vi "Inverse Time Curves (Formula, Dependent Reset).vi"(6 "operate time compensation":cluster{"G/Gs":dbl, "compensation [s]":dbl}[](array[cluster]), 7 "GD (25)":u16=25, 8 "error in (no error)":errorcluster, 9 "reset time parameters":T2={"tr [s]"=1.0, "alpha"=1.0}, 10 "time multiplier setting (1)":dbl=1.0, 11 "operate time parameters":T1={"A [s]"=1.0, "B [s]"=1.0, "alpha"=1.0, "K2 [s]"=1.0, "K1 [s]"=1.0, "K3 [s]"=1.0}) -> (0 "error out":errorcluster, 2 "memory size":u16, 3 "memory initial values":fxp<+,51,51>[](array[numeric]), 4 "curve data":cluster{"G/Gs":dbl[], "times [s]":dbl[]})   [LabVIEW 2014, in "NI_EP_Protection.lvlib"]
doc: "Generates memory initial values and memory size, which contain the information of the inverse time curves, for the FPGA Inverse Time Delay VI to use. You can compensate for the processing delay of the input energizing quantity under a specific G/Gs to achieve higher operate time accuracy."
uses:
  <vilib>/addons/Electrical Power/Protection/NI_EP_Protection.lvlib
  <vilib>/addons/Electrical Power/Protection/Inverse Time Delay/subVIs/ep_Reset Time.ctl
  <vilib>/addons/Electrical Power/Protection/Inverse Time Delay/subVIs/ep_Operate Time.ctl
  <vilib>/addons/Electrical Power/Protection/Inverse Time Delay/subVIs/ep_Curve Parameters.ctl
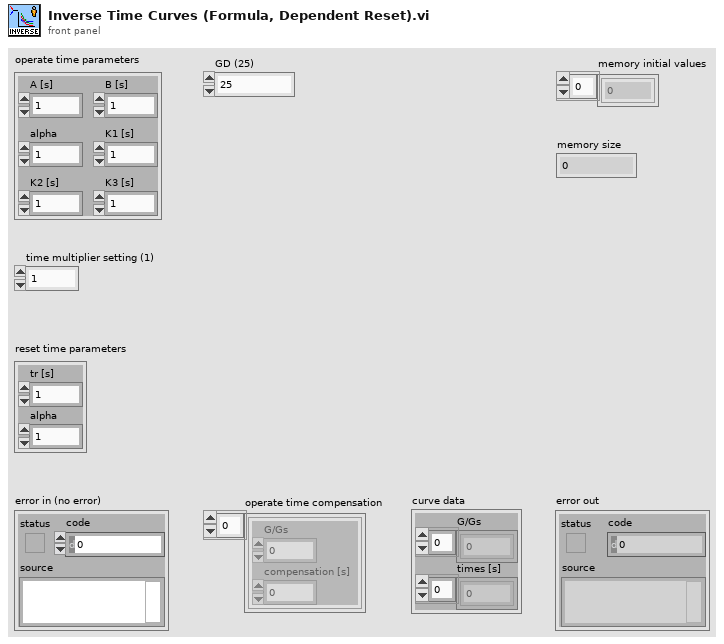
[diagram p1: front panel]
types:
  T1 = typedef "NI_EP_Protection.lvlib/ep_Operate Time.ctl" = cluster{"A [s]":dbl, "B [s]":dbl, "alpha":dbl, "K2 [s]":dbl, "K1 [s]":dbl, "K3 [s]":dbl}
  T2 = typedef "NI_EP_Protection.lvlib/ep_Reset Time.ctl" = cluster{"tr [s]":dbl, "alpha":dbl}
  T3 = typedef "NI_EP_Protection.lvlib/ep_Curve Parameters.ctl" = cluster{"operate time parameters":T1, "reset time parameters":T2}
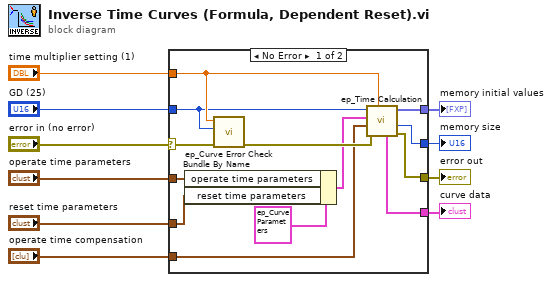
[diagram p0: block diagram]
diagram:
  n1 = case shown="No Error" "error in (no error)" {
    selector: "error in (no error)" -> [w22 w24]
    tunnel: "GD (25)" -> [w21 _]
    tunnel: "time multiplier setting (1)" -> [w23 _]
    tunnel: "operate time parameters" -> [w15 _]
    tunnel: "reset time parameters" -> [w14 _]
    tunnel: [w18 _] -> w7
    tunnel: [w19 _] -> w6
    tunnel: [w17 w24] -> w4
    tunnel: [w16 _] -> w3
    tunnel: "operate time compensation" -> [w11 _]
    frame No Error {
      n2 = Bundle By Name(cluster=T3 {"operate time parameters"={"A [s]"=1.0, "B [s]"=1.0, "alpha"=1.0, "K2 [s]"=1.0, "K1 [s]"=1.0, "K3 [s]"=1.0}, "reset time parameters"={"tr [s]"=1.0, "alpha"=1.0}} ("curve parameters"), "operate time parameters"=w15, "reset time parameters"=w14) -> (w12:T3)
      n3 = call <vilib>:"ep_Curve Error Check.vi"("error in (no error)"=w22, "GD"=w21, "time dial"=w23) -> ("error out"=w20:errorcluster)  [unwired: 8 in]
      n4 = call <vilib>:"ep_Time Calculation.vi"("time dial"=w23, "error in (no error)"=w20, "operate time compensation"=w11, "curve parameters"=w12, "GD"=w21) -> ("error out"=w17:errorcluster, "memory size"=w19:u16, "memory initial values"=w18:fxp<+,51,51>[], "curve data"=w16:cluster{"G/Gs":dbl[], "times":dbl[]})  [unwired: 3 in]
    }
    frame Error {
    }
  }
  "memory initial values" <- w7
  "memory size" <- w6
  "error out" <- w4
  "curve data" <- w3
